vi "NT_Convert Variant to NT Cluster.vi"(7 "NT_Type":T1 items=["NT_Unassigned"=0, "NT_Boolean"=1, "NT_Double"=2, "NT_String"=4, "NT_Raw"=8, "NT_BooleanArray"=16, "NT_DoubleArray"=32, "NT_StringArray"=64, "NT_RPC"=128, "NT_Integer"=256, "NT_Float"=512, "NT_IntegerArray"=1024, "NT_FloatArray"=2048], 9 "timestamp":u64, 10 "Name":string, 11 "NewVal":variant) -> (1 "NT_Type out":T1 items=["NT_Unassigned"=0, "NT_Boolean"=1, "NT_Double"=2, "NT_String"=4, "NT_Raw"=8, "NT_BooleanArray"=16, "NT_DoubleArray"=32, "NT_StringArray"=64, "NT_RPC"=128, "NT_Integer"=256, "NT_Float"=512, "NT_IntegerArray"=1024, "NT_FloatArray"=2048], 3 "Value out":variant)   [LabVIEW 2025]
doc: "Attempt to convert the LV variant type to the various NT types. If not able to do so, it may be stored as a serialized variant or become an invalid NT v ariable."
uses:
  <vilib>/Rock Robotics/Network Tables/NT Datatype.ctl
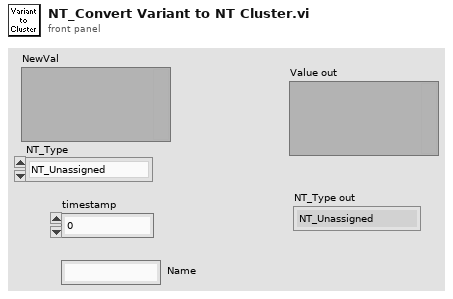
[diagram p1: front panel]
types:
  T1 = typedef "NT Datatype.ctl" = u32
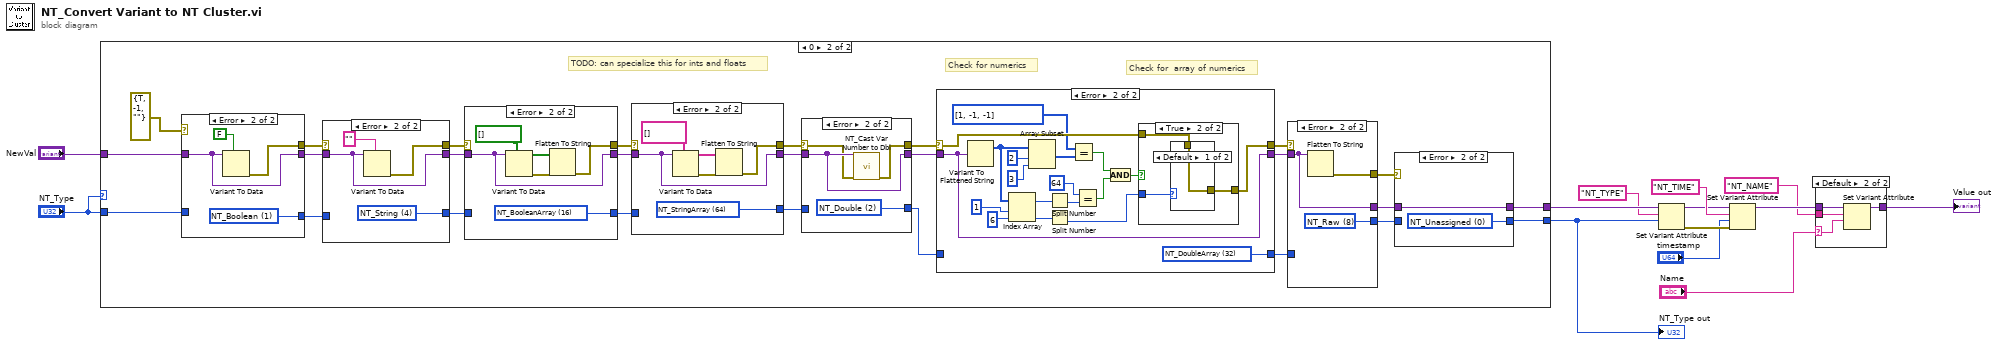
[diagram p0: block diagram]
diagram:
  n1 = case shown="0" "NT_Type" {
    tunnel: "NewVal" -> [w14 w35]
    tunnel: "NT_Type" -> [w15 w27]
    tunnel: [w14 w18] -> w12
    tunnel: [w15 w17] -> w10
    frame Default {
    }
    frame 0 {
      # "TODO: can specialize this for ints and floats"
      # "Check for  array of numerics"
      # "Check for numerics"
      n2 = case shown="Error" errorcluster {"status"=TRUE, "code"=-1, "source"=""} ("error constant") {
        selector: errorcluster {"status"=TRUE, "code"=-1, "source"=""} ("error constant") -> [w44 _]
        tunnel: w35 -> [w43 w47]
        tunnel: [w44 w48] -> w37
        tunnel: [w43 w47] -> w36
        tunnel: w27 -> [w42 _]
        tunnel: [w42 w45] -> w26
        frame No Error {
        }
        frame Error {
          w45 = T1 1 items=["NT_Unassigned"=0, "NT_Boolean"=1, "NT_Double"=2, "NT_String"=4, "NT_Raw"=8, "NT_BooleanArray"=16, "NT_DoubleArray"=32, "NT_StringArray"=64, "NT_RPC"=128, "NT_Integer"=256, "NT_Float"=512, "NT_IntegerArray"=1024, "NT_FloatArray"=2048] ("NT_Type")
          n3 = Variant To Data(type=FALSE ("status"), Variant=w47) -> (error out=w48:errorcluster)  [unwired: 1 in, 1 out]
        }
      }
      n4 = case shown="Error" w37 {
        selector: w37 -> [w51 _]
        tunnel: w36 -> [w50 w53]
        tunnel: [w51 w54] -> w41
        tunnel: [w50 w53] -> w40
        tunnel: [w49 w52] -> w25
        tunnel: w26 -> [w49 _]
        frame No Error {
        }
        frame Error {
          w52 = T1 4 items=["NT_Unassigned"=0, "NT_Boolean"=1, "NT_Double"=2, "NT_String"=4, "NT_Raw"=8, "NT_BooleanArray"=16, "NT_DoubleArray"=32, "NT_StringArray"=64, "NT_RPC"=128, "NT_Integer"=256, "NT_Float"=512, "NT_IntegerArray"=1024, "NT_FloatArray"=2048] ("NT_Type")
          n5 = Variant To Data(type="", Variant=w53) -> (error out=w54:errorcluster)  [unwired: 1 in, 1 out]
        }
      }
      n6 = case shown="Error" w41 {
        selector: w41 -> [w58 _]
        tunnel: w40 -> [w57 w64]
        tunnel: [w58 w60] -> w39
        tunnel: [w57 w64] -> w38
        tunnel: [w56 w59] -> w24
        tunnel: w25 -> [w56 _]
        frame No Error {
        }
        frame Error {
          w59 = T1 16 items=["NT_Unassigned"=0, "NT_Boolean"=1, "NT_Double"=2, "NT_String"=4, "NT_Raw"=8, "NT_BooleanArray"=16, "NT_DoubleArray"=32, "NT_StringArray"=64, "NT_RPC"=128, "NT_Integer"=256, "NT_Float"=512, "NT_IntegerArray"=1024, "NT_FloatArray"=2048] ("NT_Type")
          n7 = Variant To Data(type=bool[] [], Variant=w64) -> (data=w61:bool[], error out=w62:errorcluster)  [unwired: 1 in]
          n8 = Flatten To String(anything=w61, error in (no error)=w62) -> (error out=w60:errorcluster)  [unwired: 2 in, 2 out]
        }
      }
      n9 = case shown="Error" w39 {
        selector: w39 -> [w67 _]
        tunnel: w38 -> [w66 w73]
        tunnel: [w67 w70] -> w34
        tunnel: [w66 w73] -> w33
        tunnel: [w65 w68] -> w23
        tunnel: w24 -> [w65 _]
        frame No Error {
        }
        frame Error {
          w68 = T1 64 items=["NT_Unassigned"=0, "NT_Boolean"=1, "NT_Double"=2, "NT_String"=4, "NT_Raw"=8, "NT_BooleanArray"=16, "NT_DoubleArray"=32, "NT_StringArray"=64, "NT_RPC"=128, "NT_Integer"=256, "NT_Float"=512, "NT_IntegerArray"=1024, "NT_FloatArray"=2048] ("NT_Type")
          n10 = Variant To Data(type=string[] [], Variant=w73) -> (data=w71:string[], error out=w72:errorcluster)  [unwired: 1 in]
          n11 = Flatten To String(anything=w71, error in (no error)=w72) -> (error out=w70:errorcluster)  [unwired: 2 in, 2 out]
        }
      }
      n12 = case shown="Error" w34 {
        selector: w34 -> [w76 w78]
        tunnel: w33 -> [w75 w80]
        tunnel: [w76 w79] -> w32
        tunnel: [w75 w80] -> w31
        tunnel: [w74 w77] -> w22
        tunnel: w23 -> [w74 _]
        frame No Error {
        }
        frame Error {
          w77 = T1 2 items=["NT_Unassigned"=0, "NT_Boolean"=1, "NT_Double"=2, "NT_String"=4, "NT_Raw"=8, "NT_BooleanArray"=16, "NT_DoubleArray"=32, "NT_StringArray"=64, "NT_RPC"=128, "NT_Integer"=256, "NT_Float"=512, "NT_IntegerArray"=1024, "NT_FloatArray"=2048] ("NT_Type")
          n13 = call <vilib>:"NT_Cast Var Number to Dbl.vi"("error in (no error)"=w78, "NewVal"=w80) -> ("error out"=w79:errorcluster)  [unwired: 8 in, 1 out]
        }
      }
      n14 = case shown="Error" w32 {
        selector: w32 -> [w83 w99]
        tunnel: w31 -> [w82 w101]
        tunnel: [w83 w100] -> w29
        tunnel: [w82 w101] -> w30
        tunnel: [w81 w84] -> w21
        tunnel: w22 -> [w81 _]
        frame No Error {
        }
        frame Error {
          w84 = T1 32 items=["NT_Unassigned"=0, "NT_Boolean"=1, "NT_Double"=2, "NT_String"=4, "NT_Raw"=8, "NT_BooleanArray"=16, "NT_DoubleArray"=32, "NT_StringArray"=64, "NT_RPC"=128, "NT_Integer"=256, "NT_Float"=512, "NT_IntegerArray"=1024, "NT_FloatArray"=2048] ("NT_Type")
          n15 = Variant To Flattened String(Variant=w101) -> (1:w95:i16[])  [unwired: 1 out]
          n16 = Index Array(array=w95, index #1=1 ("index"), index #2=6 ("index")) -> (element #1=w90:i16, element #2=w93:i16)
          n17 = Array Subset(array=w95, index=2, length=3 ("index")) -> (w97:i16[])
          n18 = Split Number(x=w90) -> (lo(x)=w89:u8)  [unwired: 1 out]
          n19 = Split Number(x=w93) -> (lo(x)=w92:u8)  [unwired: 1 out]
          n20 = Equal?(x=i16[] [1, -1, -1], y=w97) -> (x = y?=w86:bool)
          n21 = Equal?(x=i16 64 ("index"), y=w89) -> (x = y?=w85:bool)
          n22 = And(x=w86, y=w85) -> (x .and. y?=w87:bool)
          n23 = case shown="True" w87 {
            tunnel: [w103 w106] -> w100
            tunnel: w99 -> [w103 w105]
            tunnel: w92 -> [_ w104]
            frame False {
            }
            frame True {
              n24 = case shown="Default" w104 {
                tunnel: [w107 _] -> w106
                tunnel: w105 -> [w107 _]
                frame Default {
                }
                frame 1..11 {
                }
              }
            }
          }
        }
      }
      n25 = case shown="Error" w29 {
        selector: w29 -> [w110 _]
        tunnel: w30 -> [w108 w111]
        tunnel: [w110 w113] -> w28
        tunnel: [w109 w112] -> w20
        tunnel: w21 -> [w109 _]
        tunnel: [w108 w111] -> w19
        frame No Error {
        }
        frame Error {
          w112 = T1 8 items=["NT_Unassigned"=0, "NT_Boolean"=1, "NT_Double"=2, "NT_String"=4, "NT_Raw"=8, "NT_BooleanArray"=16, "NT_DoubleArray"=32, "NT_StringArray"=64, "NT_RPC"=128, "NT_Integer"=256, "NT_Float"=512, "NT_IntegerArray"=1024, "NT_FloatArray"=2048] ("NT_Type")
          n26 = Flatten To String(anything=w111) -> (error out=w113:errorcluster)  [unwired: 3 in, 2 out]
        }
      }
      n27 = case shown="Error" w28 {
        tunnel: [w115 w117] -> w17
        tunnel: w20 -> [w115 _]
        tunnel: [w114 w116] -> w18
        tunnel: w19 -> [w114 w116]
        frame No Error {
        }
        frame Error {
          w117 = T1 0 items=["NT_Unassigned"=0, "NT_Boolean"=1, "NT_Double"=2, "NT_String"=4, "NT_Raw"=8, "NT_BooleanArray"=16, "NT_DoubleArray"=32, "NT_StringArray"=64, "NT_RPC"=128, "NT_Integer"=256, "NT_Float"=512, "NT_IntegerArray"=1024, "NT_FloatArray"=2048] ("NT_Type")
        }
      }
    }
  }
  "NT_Type out" <- w10
  n28 = Set Variant Attribute(Variant=w12, name="NT_TYPE" ("String"), value=w10) -> (Variant out=w8:variant, error out=w7:errorcluster)  [unwired: 1 in, 1 out]
  n29 = Set Variant Attribute(Variant=w8, name="NT_TIME" ("String"), value="timestamp", error in=w7) -> (Variant out=w5:variant)  [unwired: 2 out]
  n30 = case shown="Default" "Name" {
    selector: "Name" -> [_ w119]
    tunnel: w5 -> [w118 w122]
    tunnel: [w118 w121] -> w4
    tunnel: "NT_NAME" ("String") -> [_ w120]
    frame "" {
    }
    frame Default {
      n31 = Set Variant Attribute(Variant=w122, name=w120, value=w119) -> (Variant out=w121:variant)  [unwired: 1 in, 2 out]
    }
  }
  "Value out" <- w4
